vi "Set Queue Service Properties.vi"(8 "error in (no error)":errorcluster, 10 "Queue Service Properties":T1, 11 "Azure Session in":refnum<class "Session.lvclass">) -> (0 "error out":errorcluster, 3 "Azure Session out":refnum<class "Session.lvclass">)   [LabVIEW 2015, in "NI_Azure_Queue.lvlib"]
doc: "Sets the properties of the Queue service."
uses:
  NI_Azure_Queue.lvlib
  Core/Session/Session.lvclass
  Queue Service Properties.ctl
  Logging.ctl
  Retention Policy.ctl
  Metrics.ctl
  Cors Rule.ctl
  Core/Name Value Pair.ctl
  Core/Session/Session.lvclass/Session.ctl
  Core/Session/Write Request Parameters.vi
  Core/Session/Write Request body.vi
  Core/Session/Write HTTP Verb.vi
  Core/NI_Azure_Core.lvlib
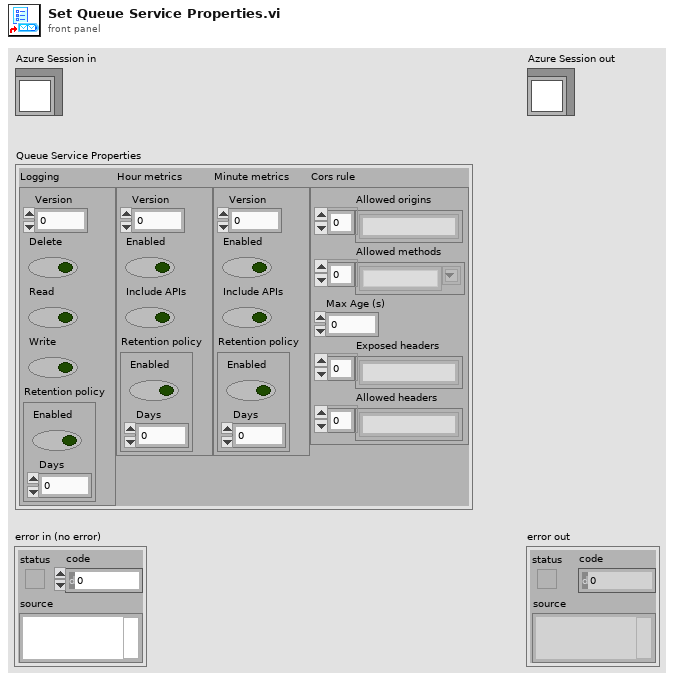
[diagram p1: front panel]
types:
  T1 = typedef "NI_Azure_Queue.lvlib/Queue Service Properties.ctl" = cluster{"Logging":T2, "Hour metrics":T4, "Minute metrics":T4, "Cors rule":T5}
  T2 = typedef "NI_Azure_Queue.lvlib/Logging.ctl" = cluster{"Version":dbl, "Delete":bool, "Read":bool, "Write":bool, "Retention policy":T3}
  T3 = typedef "NI_Azure_Queue.lvlib/Retention Policy.ctl" = cluster{"Enabled":bool, "Days":u32}
  T4 = typedef "NI_Azure_Queue.lvlib/Metrics.ctl" = cluster{"Version":dbl, "Enabled":bool, "Include APIs":bool, "Retention policy":T3}
  T5 = typedef "NI_Azure_Queue.lvlib/Cors Rule.ctl" = cluster{"Allowed origins":string[], "Allowed methods":string[], "Max Age (s)":u32, "Exposed headers":string[], "Allowed headers":string[]}
  T6 = typedef "NI_Azure_Core.lvlib/Name Value Pair.ctl" = cluster{"name":string, "value":string}
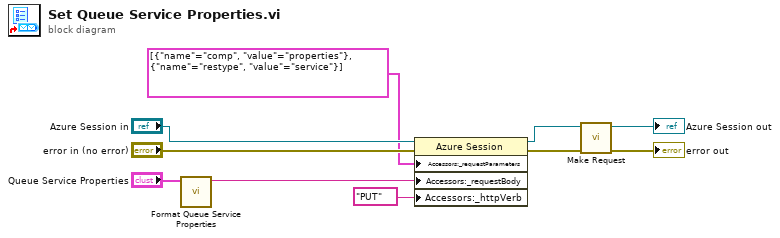
[diagram p0: block diagram]
diagram:
  n1 = call "Format Queue Service Properties.vi"("Queue service properties"="Queue Service Properties") -> ("Queue service string"=w3:string)  [unwired: 10 in]
  n2 = property class="Azure Session"(reference="Azure Session in", error in="error in (no error)", "Accessors:_requestParameters"=T6[] [{"name"="comp", "value"="properties"}, {"name"="restype", "value"="service"}] ("request parameters"), "Accessors:_requestBody"=w3, "Accessors:_httpVerb"="PUT" ("HTTP-Verb")) -> (reference out=w4:refnum<class "Session.lvclass">, error out=w6:errorcluster)
  n3 = call "Make Request.vi"("error in (no error)"=w6, "Session in"=w4) -> ("error out"=→"error out":errorcluster, "Session out"=→"Azure Session out":refnum<class "Session.lvclass">)  [unwired: 7 in, 1 out]
